vi "模拟量配置.vi"(11 "工程量转换":T2={"原始值最小值"=0.0, "原始值最大值"=1.0, "转换值最小值"=0.0, "转换值最大值"=1.0, "原始值最小值 2"=0.0, "原始值最大值 2"=1.0, "转换值最小值 2"=0.0, "转换值最大值 2"=1.0, "原始值最小值 3"=0.0, "原始值最大值 3"=1.0, "转换值最小值 3"=0.0, "转换值最大值 3"=1.0, "原始值最小值 4"=0.0, "原始值最大值 4"=1.0, "转换值最小值 4"=0.0, "转换值最大值 4"=1.0, "原始值最小值 5"=0.0, "原始值最大值 5"=1.0, "转换值最小值 5"=0.0, "转换值最大值 5"=1.0, "原始值最小值 6"=0.0, "原始值最大值 6"=1.0, "转换值最小值 6"=0.0, "转换值最大值 6"=1.0, "原始值最小值 7"=0.0, "原始值最大值 7"=1.0, "转换值最小值 7"=0.0, "转换值最大值 7"=1.0, "原始值最小值 8"=0.0, "原始值最大值 8"=1.0, "转换值最小值 8"=0.0, "转换值最大值 8"=1.0} {"转换值最大值 8" format="%#.2f"; "转换值最小值 8" format="%#.2f"; "原始值最大值 8" format="%#.2f"; "原始值最小值 8" format="%#.2f"; "转换值最大值 7" format="%#.2f"; "转换值最小值 7" format="%#.2f"; "原始值最大值 7" format="%#.2f"; "原始值最小值 7" format="%#.2f"; "转换值最大值 6" format="%#.2f"; "转换值最小值 6" format="%#.2f"; "原始值最大值 6" format="%#.2f"; "原始值最小值 6" format="%#.2f"; "转换值最大值 5" format="%#.2f"; "转换值最小值 5" format="%#.2f"; "原始值最大值 5" format="%#.2f"; "原始值最小值 5" format="%#.2f"; "转换值最大值 4" format="%#.2f"; "转换值最小值 4" format="%#.2f"; "原始值最大值 4" format="%#.2f"; "原始值最小值 4" format="%#.2f"; "转换值最大值 3" format="%#.2f"; "转换值最小值 3" format="%#.2f"; "原始值最大值 3" format="%#.2f"; "原始值最小值 3" format="%#.2f"; "转换值最大值 2" format="%#.2f"; "转换值最小值 2" format="%#.2f"; "原始值最大值 2" format="%#.2f"; "原始值最小值 2" format="%#.2f"; "转换值最大值" format="%#.2f"; "转换值最小值" format="%#.2f"; "原始值最大值" format="%#.2f"; "原始值最小值" format="%#.2f"}) -> ()   [LabVIEW 2016, in "采配水.lvlib"]
uses:
  <vilib>/Utility/miscctls.llb/LVPointTypeDef.ctl
  <vilib>/Utility/config.llb/NI_LVConfig.lvlib
panel:
  out "工程值":T1 {"AD7" format="%.2f"; "AD6" format="%.2f"; "AD5" format="%.2f"; "AD4" format="%.2f"; "AD3" format="%.2f"; "AD2" format="%.2f"; "AD1" format="%.2f"; "AD0" format="%.2f"}
  out "当前值":T1 {"AD7" format="%.2f"; "AD6" format="%.2f"; "AD5" format="%.2f"; "AD4" format="%.2f"; "AD3" format="%.2f"; "AD2" format="%.2f"; "AD1" format="%.2f"; "AD0" format="%.2f"}
  in  "关闭":bool
  in  "应用":bool
  # "当前原始值："
  # "工程值："
  # "原始低值"
  # "原始高值"
  # "转换低值"
  # "转换高值"
  # "AD7:"
  # "AD6:"
  # "AD5:"
  # "AD4:"
  # "AD3:"
  # "AD2:"
  # "AD1:"
  # "AD0:"
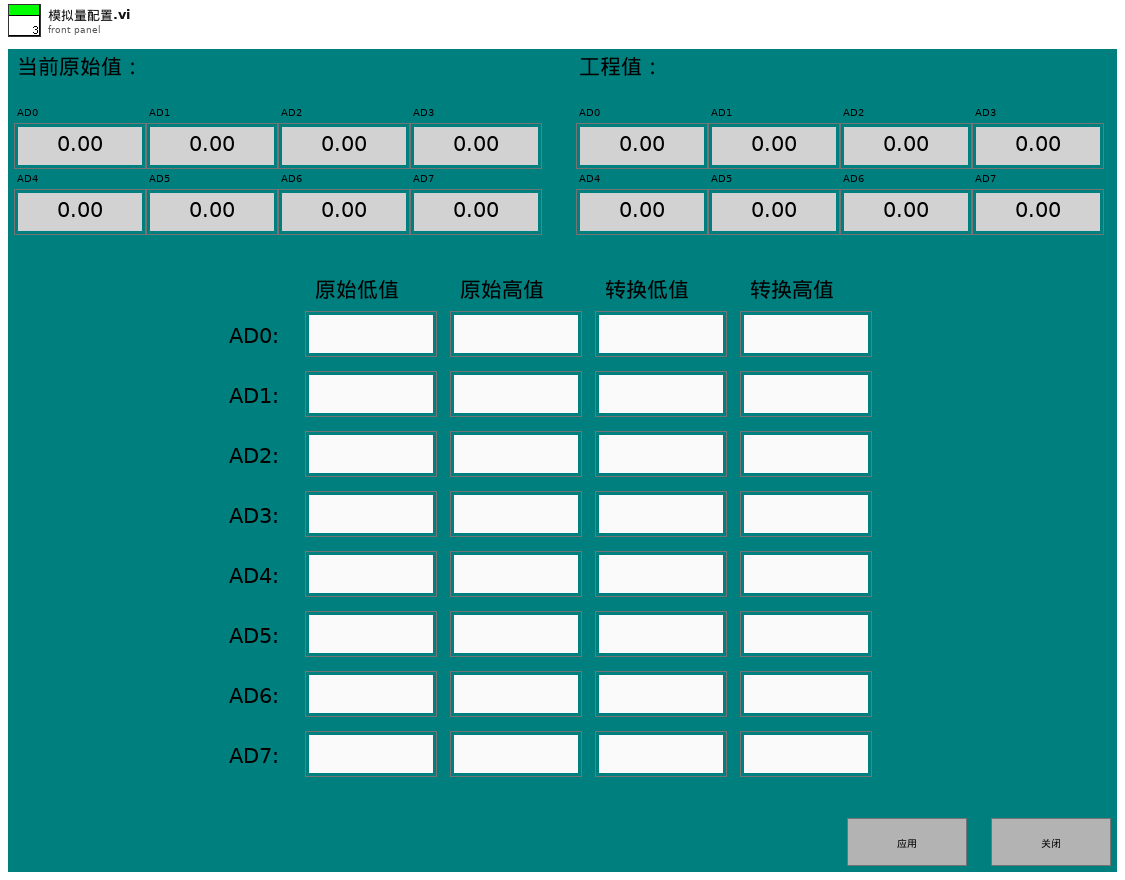
[diagram p1: front panel]
types:
  T1 = cluster{"AD0":dbl, "AD1":dbl, "AD2":dbl, "AD3":dbl, "AD4":dbl, "AD5":dbl, "AD6":dbl, "AD7":dbl}
  T2 = cluster{"原始值最小值":dbl, "原始值最大值":dbl, "转换值最小值":dbl, "转换值最大值":dbl, "原始值最小值 2":dbl, "原始值最大值 2":dbl, "转换值最小值 2":dbl, "转换值最大值 2":dbl, "原始值最小值 3":dbl, "原始值最大值 3":dbl, "转换值最小值 3":dbl, "转换值最大值 3":dbl, "原始值最小值 4":dbl, "原始值最大值 4":dbl, "转换值最小值 4":dbl, "转换值最大值 4":dbl, "原始值最小值 5":dbl, "原始值最大值 5":dbl, "转换值最小值 5":dbl, "转换值最大值 5":dbl, "原始值最小值 6":dbl, "原始值最大值 6":dbl, "转换值最小值 6":dbl, "转换值最大值 6":dbl, "原始值最小值 7":dbl, "原始值最大值 7":dbl, "转换值最小值 7":dbl, "转换值最大值 7":dbl, "原始值最小值 8":dbl, "原始值最大值 8":dbl, "转换值最小值 8":dbl, "转换值最大值 8":dbl}
  T3 = typedef "LVPointTypeDef.ctl" = cluster{"Horizontal":i16, "Vertical":i16}
  T4 = cluster{"AD0":dbl, "AD1":dbl, "AD1":dbl, "AD3":dbl, "AD4":dbl, "AD5":dbl, "AD6":dbl, "AD7":dbl}
  T5 = typedef "NI_LVConfig.lvlib/Config Data RefNum.ctl" = refnum<k1>
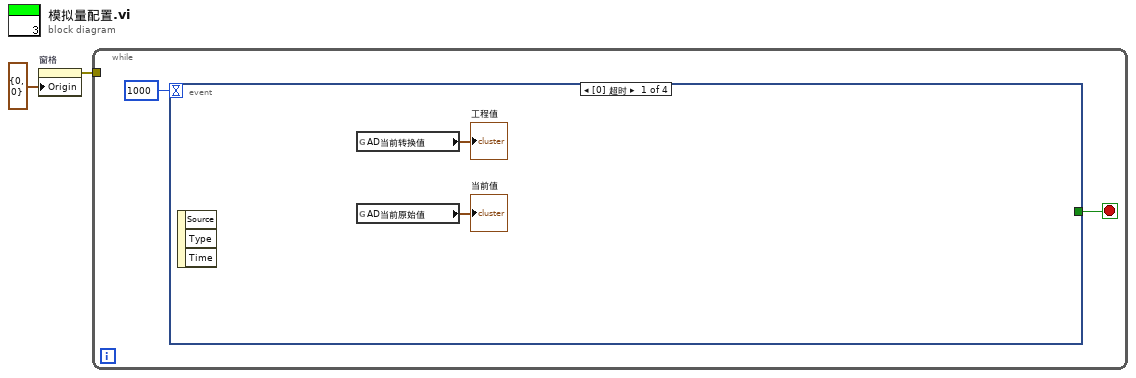
[diagram p0: block diagram]
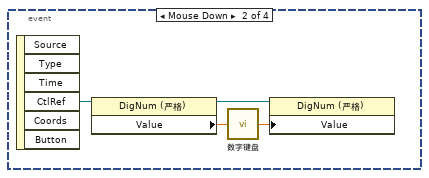
[diagram p2: hidden frame]
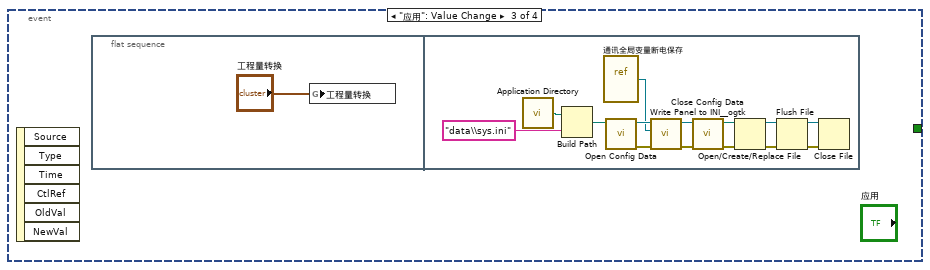
[diagram p3: hidden frame]
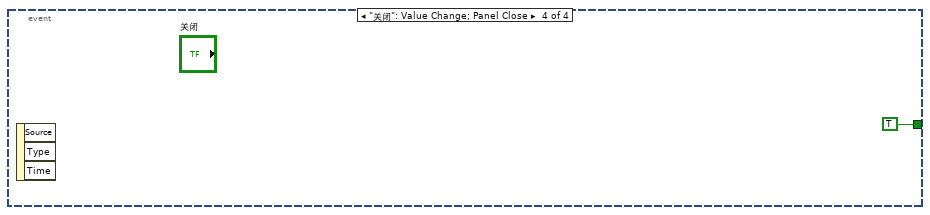
[diagram p4: hidden frame]
diagram:
  n1 = property on="窗格" class="Pane"("Origin"=T3 {"Horizontal"=0, "Vertical"=0} ("原点")) -> (error out=w1:errorcluster)  [unwired: 2 in, 1 out]
  n2 = while {
    tunnel: w1 -> [_]
    stop <- w3 stop-if-true
    n3 = event shown="[0] 超时" {
      selector: _ -> [_ _ _ _]
      dyn-events: _ -> [_ _ _ _]
      timeout: 1000 -> [_ _ _ _]
      tunnel: [_ _ _ TRUE] -> w3
      event Timeout {
        n4 = event-data() -> ()  [unwired: 1 in, 3 out]
        n5 = global read "通讯全局变量.vi" "AD当前转换值"() -> (→"工程值":T1)
        n6 = global read "通讯全局变量.vi" "AD当前原始值"() -> (→"当前值":T4)
      }
      event "工程量转换.原始值最小值", "工程量转换.原始值最大值", "工程量转换.转换值最小值", "工程量转换.转换值最大值", "工程量转换.转换值最大值 2", "工程量转换.转换值最小值 2", "工程量转换.原始值最大值 2", "工程量转换.原始值最小值 2", "工程量转换.转换值最大值 3", "工程量转换.转换值最小值 3", "工程量转换.原始值最小值 3", "工程量转换.原始值最大值 3", "工程量转换.转换值最大值 4", "工程量转换.转换值最小值 4", "工程量转换.原始值最大值 4", "工程量转换.原始值最小值 4", "工程量转换.转换值最大值 5", "工程量转换.转换值最小值 5", "工程量转换.原始值最大值 5", "工程量转换.原始值最小值 5", "工程量转换.转换值最大值 6", "工程量转换.转换值最小值 6", "工程量转换.原始值最大值 6", "工程量转换.原始值最小值 6", "工程量转换.转换值最大值 7", "工程量转换.转换值最小值 7", "工程量转换.原始值最大值 7", "工程量转换.原始值最小值 7", "工程量转换.转换值最大值 8", "工程量转换.转换值最小值 8", "工程量转换.原始值最大值 8", "工程量转换.原始值最小值 8": Mouse Down {
        n7 = event-data() -> ("CtlRef"=w10:refnum<vi>)  [unwired: 1 in, 5 out]
        n8 = property class="DigNum (严格)"(reference=w10) -> (reference out=w8:refnum<vi>, "Value"=w9:dbl)  [unwired: 1 in, 1 out]
        n9 = call "数字键盘.vi"("OldNumber"=w9) -> ("NewNumber"=w7:dbl)
        n10 = property class="DigNum (严格)"(reference=w8, "Value"=w7) -> ()  [unwired: 1 in, 2 out]
      }
      event "应用": Value Change {
        n11 = event-data() -> ()  [unwired: 1 in, 6 out]
        n12 = flat-sequence {
          frame #0 {
            n13 = global write "通讯全局变量断电保存.vi" "工程量转换"("工程量转换") -> ()
          }
          frame #1 {
            n14 = call <vilib>:"Application Directory.vi"() -> ("Application Directory"=w25:path)
            n15 = Build Path(base path=w25, name or relative path="data\\sys.ini" ("名称或相对路径")) -> (appended path=w23:path)
            n16 = vi-ref "通讯全局变量断电保存.vi"() -> (w21:refnum<vi>)
            n17 = call <vilib>:"Open Config Data.vi"("configuration file path"=w23) -> ("error out"=w19:errorcluster, "refnum"=w22:T5)  [unwired: 8 in, 1 out]
            n18 = call <userlib>:"Write Panel to INI__ogtk.vi"("error in (no error)"=w19, "VI ref"=w21, "refnum"=w22) -> ("error out"=w18:errorcluster, "refnum out"=w20:T5)  [unwired: 7 in]
            n19 = call <vilib>:"Close Config Data.vi"("error in (no error)"=w18, "refnum"=w20) -> ("error out"=w13:errorcluster, "file path"=w12:path)  [unwired: 8 in]
            n20 = Open/Create/Replace File(file path (use dialog)=w12, error in=w13) -> (refnum out=w16:refnum<file>, error out=w17:errorcluster)  [unwired: 4 in, 1 out]
            n21 = Flush File(refnum=w16, error in=w17) -> (refnum out=w15:refnum<file>, error out=w14:errorcluster)
            n22 = Close File(refnum=w15, error in=w14) -> ()  [unwired: 2 out]
          }
        }
      }
      event "关闭": Value Change; Panel Close {
        n23 = event-data() -> ()  [unwired: 1 in, 3 out]
      }
    }
  }
